vi "Update_Single_Log_Table_pibs.vi"(6 "String":string, 7 "tableIndx":i32 caption="Which Log Table", 8 "colIndx":i32 caption="Which Col Index", 9 "insertRow":i32, 10 "pass8thRow":bool, 11 "logTable in":string[][][](array[string])) -> (3 "logTable out":string[][][](array[string]))   [LabVIEW 2013]
panel:
  out "logTableOutNew":string[][](array[string])
  out "logTableOut":string[][](array[string])
  out "logTableIn":string[][](array[string])
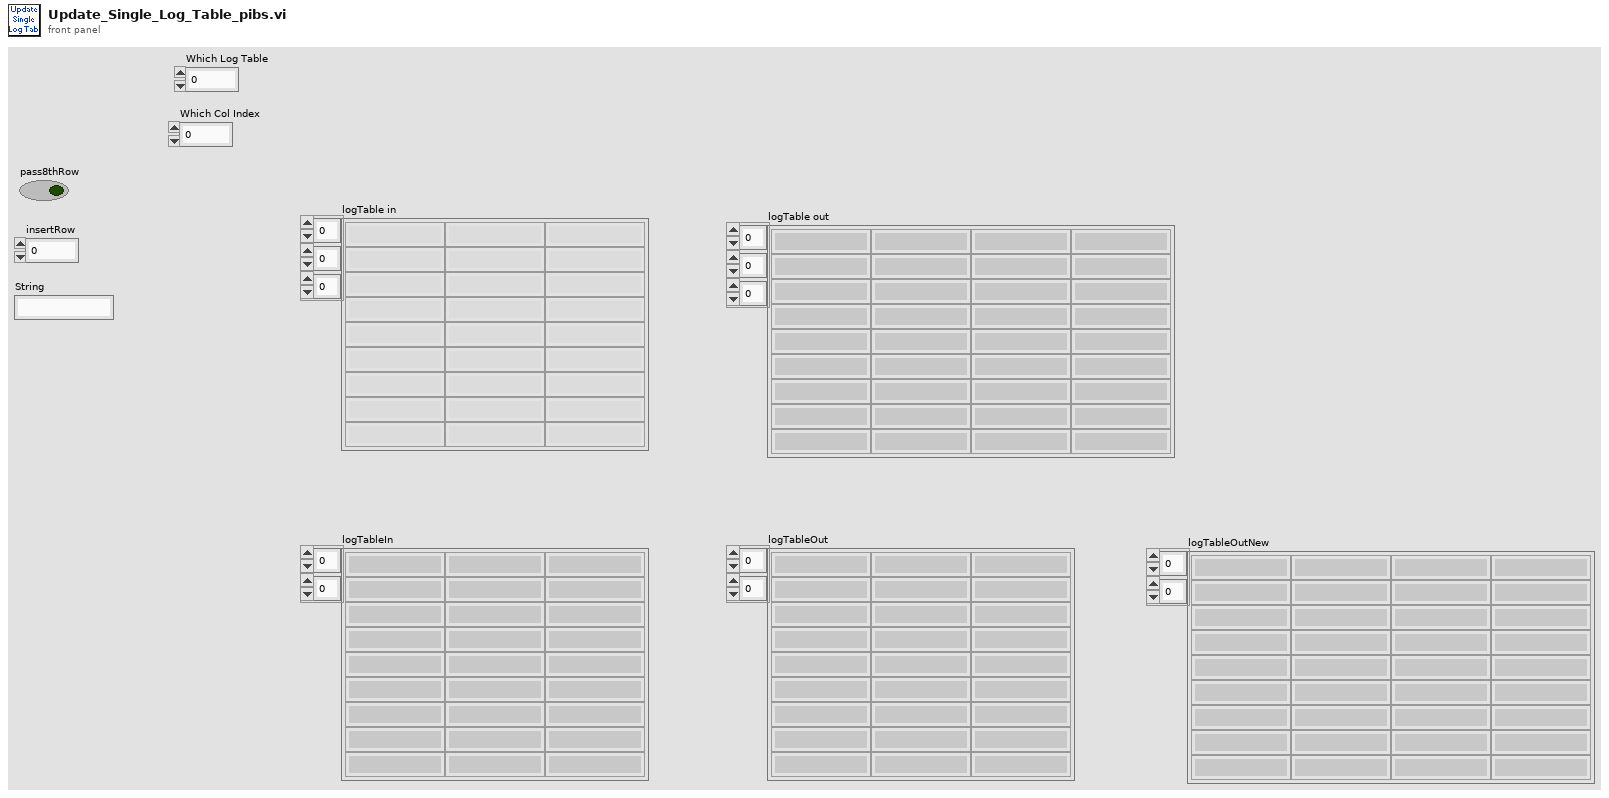
[diagram p1: front panel]
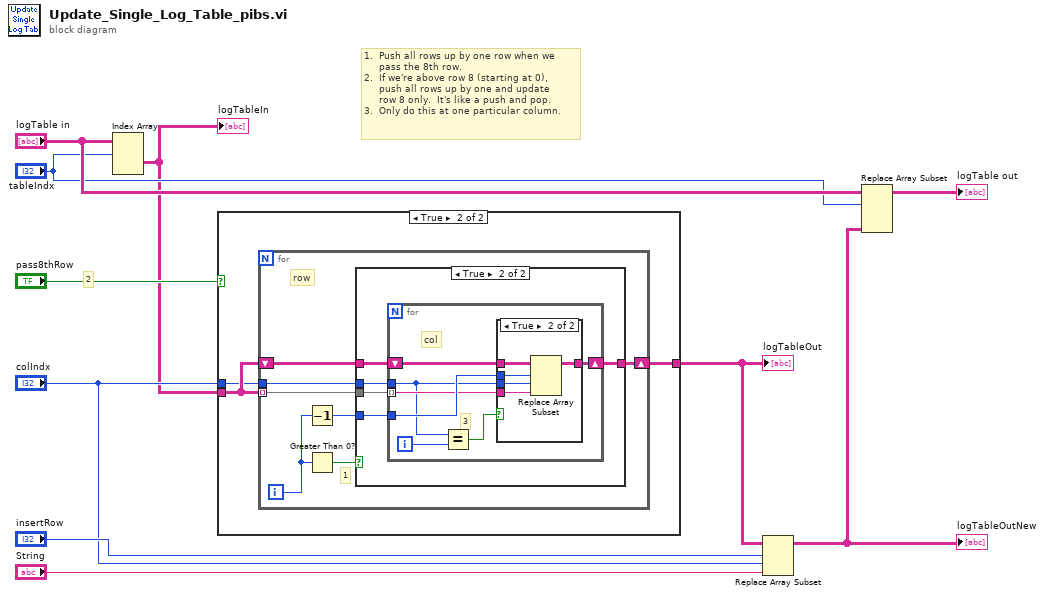
[diagram p0: block diagram]
diagram:
  # "2"
  # "1.  Push all rows up by one row when we\n     pass the 8th row.\n2.  If we're above row 8 (starting at 0),\n     push all rows up by one and update\n     row 8 only.  It's like a push and pop.\n3.  Only do this at one particular column."
  n1 = Index Array(array="logTable in", index (dim 0)="tableIndx") -> (element=w1:string[][])  [unwired: 2 in]
  "logTableIn" <- w1
  n2 = case shown="True" "pass8thRow" {
    tunnel: w1 -> [w11 w14]
    tunnel: [w11 w13] -> w6
    tunnel: "colIndx" -> [_ w12]
    frame False {
    }
    frame True {
      n3 = for {
        tunnel: w14 -> [w20] mode=indexing
        shift-right: [w19] -> w13
        shift-left: w14 -> [w21]
        tunnel: w12 -> [w18]
        i -> [w17]
        # "1"
        # "row"
        n4 = Decrement(x=w17) -> (x-1=w15:i32)
        n5 = Greater Than 0?(x=w17) -> (x > 0?=w16:bool)
        n6 = case shown="True" w16 {
          tunnel: w21 -> [w22 w27]
          tunnel: w20 -> [_ w26]
          tunnel: [w22 w25] -> w19
          tunnel: w18 -> [_ w24]
          tunnel: w15 -> [_ w23]
          frame False {
          }
          frame True {
            n7 = for {
              tunnel: w26 -> [w30] mode=indexing
              tunnel: w24 -> [w29]
              shift-right: [w33] -> w25
              shift-left: w27 -> [w34]
              tunnel: w23 -> [w31]
              i -> [w32]
              # "3"
              # "col"
              n8 = Equal?(x=w29, y=w32) -> (x = y?=w28:bool)
              n9 = case shown="True" w28 {
                tunnel: w34 -> [w35 w40]
                tunnel: [w35 w39] -> w33
                tunnel: w31 -> [_ w38]
                tunnel: w30 -> [_ w37]
                tunnel: w29 -> [_ w36]
                frame False {
                }
                frame True {
                  n10 = Replace Array Subset(array=w40, new element=w37, index (row)=w38, index (col)=w36) -> (w39:string[][])
                }
              }
            }
          }
        }
      }
    }
  }
  "logTableOut" <- w6
  n11 = Replace Array Subset(array=w6, new element="String", index (row)="insertRow", index (col)="colIndx") -> (w5:string[][])
  "logTableOutNew" <- w5
  n12 = Replace Array Subset(array="logTable in", new element=w5, index (dim 0)="tableIndx") -> (→"logTable out":string[][][])  [unwired: 2 in]
